vi "Data output .vi"(0 "Cluster in":refnum<vi>, 1 "Knob Refnum":refnum<vi>, 2 "Output data format":T1(ring), 5 "Pict Refnum":refnum<vi>, 7 "Clust Refnum in":refnum<vi>, 9 "Clust Refnum 3":refnum<vi>, 12 "String":string, 13 "Gyro rande \n(deg/sec)":T2(ring), 14 "Accel range \n(g)":enum16{"2", "4", "6", "8", "10", "15", "40"}(ring)) -> (3 "Gauge":i32(knob) scale=0.0..360.0, 4 "2D Picture":picture, 6 "Cluster":T5 {"Altitude" format="%#_11g"; "Longitude" format="%#_11g"; "Latitude" format="%#_11g"}, 8 "Sensors":T3 {"Altitude" format="%#_11g"; "Longitude" format="%#_11g"; "Latitude" format="%#_11g"}, 10 "QPVT":T4 {"Altitude" format="%#_11g"; "Longitude" format="%#_11g"; "Latitude" format="%#_11g"})   [LabVIEW 2017, in "IL Driver Library.lvlib"]
uses:
  IL Driver library.lvlib
panel:
  # "Orientation angles (deg)"
  # "Sensors output\n(ADC code)"
  # "Rate"
  # "Accel"
  # "Magn"
  # "X"
  # "Y"
  # "Z"
  # "Additional\n   (code)"
  # "Position abs (deg,m)"
  # "Quaternion of orientation"
  # "Sensors output"
  # "Rate(deg/s)"
  # "Accel(g)"
  # "Magn(nT)"
  # "X"
  # "Y"
  # "Z"
  # "Additional"
  # "Position abs (deg,m)"
  # "Orientation angles (deg)"
  # "Sensors output"
  # "Rate(deg/s)"
  # "Accel(g)"
  # "Magn(nT)"
  # "X"
  # "Y"
  # "Z"
  # "Additional"
  # "Position abs (deg,m)"
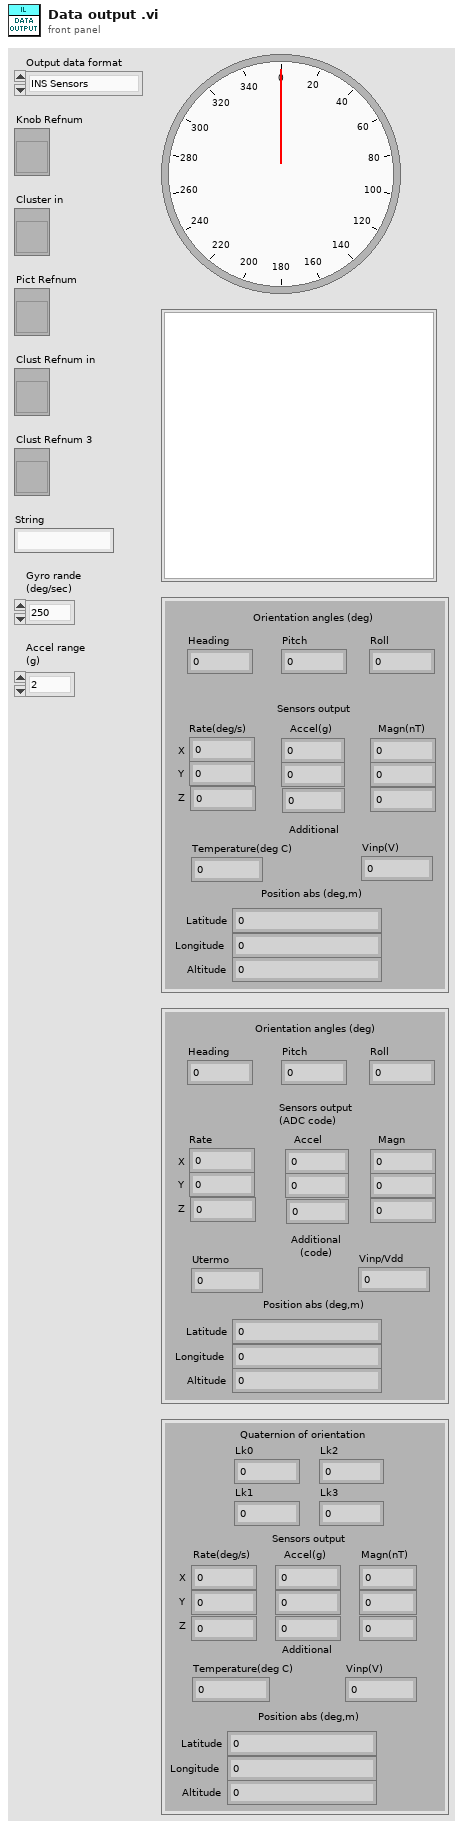
[diagram p1: front panel]
types:
  T1 = enum16{"INS Sensors", "INS OPVT", "INS QPVT", "INS OPVT2A", "INS OPVT2AW", "INS OPVT2Ahr", "INS Minimal", "INS NMEA"}
  T2 = enum16{"250", "300", "450", "500", "1000", "2000"}
  T3 = cluster{"Heading":dbl, "Pitch":dbl, "Roll":dbl, "GyroX(deg/s)":dbl, "GyroY(deg/s)":dbl, "GyroZ(deg/s)":dbl, "AxelX(g)":dbl, "AxelY(g)":dbl, "AxelZ(g)":dbl, "Dec":i32, "MagY":i32, "MagZ":i32, "Utermo":dbl, "Vinp/Vdd":dbl, "Latitude":dbl, "Longitude":dbl, "Altitude":dbl}
  T4 = cluster{"Lk0":dbl, "Lk1":dbl, "Lk2":dbl, "Lk3":dbl, "Numeric 5":dbl, "Numeric 6":dbl, "Numeric 7":dbl, "Numeric 8":dbl, "Numeric 9":dbl, "Numeric 10":dbl, i32, i32, i32, "Temperature(deg C)":dbl, "Vinp(V)":dbl, "Latitude":dbl, "Longitude":dbl, "Altitude":dbl}
  T5 = cluster{"Heading":dbl, "Pitch":dbl, "Roll":dbl, "GyroX(deg/s)":dbl, "GyroY(deg/s)":dbl, "GyroZ(deg/s)":dbl, "AxelX(g)":dbl, "AxelY(g)":dbl, "AxelZ(g)":dbl, "Dec":i32, "MagY":i32, "MagZ":i32, "Temperature(deg C)":dbl, "Vinp(V)":dbl, "Latitude":dbl, "Longitude":dbl, "Altitude":dbl}
  T6 = cluster{dbl, dbl, dbl, "Dec":i16, "Dec":i16, "Dec":i16, "Dec":i16, "Dec":i16, "Dec":i16, "Dec":i16, "Dec":i16, "Dec":i16, "Dec":i16, dbl, "Dec":u16, "Dec":u16, "Dec":i16, dbl, dbl, dbl, dbl, dbl, dbl, dbl, dbl, dbl, "Dec":i32, "Dec":u8, "Dec":u8, "Dec":u8, "Dec":u8, "Dec":u8, "Dec":u8, "Dec":u8, "Dec":u8, "Dec":u8, "Dec":u8, "Dec":u8, "Dec":u8, "Dec":u16, "Dec":u16, "Dec":u8, "Dec":u8}
  T7 = cluster{dbl, dbl, dbl, dbl, dbl, dbl, dbl, dbl, dbl, i32, i32, i32, "Dec":u16, dbl, dbl, dbl, dbl, dbl, dbl, dbl, dbl, dbl, dbl, dbl, dbl, dbl, dbl, "Dec":i32, "Dec":u8, "Dec":u8, "Dec":u8, dbl, "Dec":u16, dbl, "Dec":u8}
  T8 = cluster{dbl, dbl, dbl, dbl, dbl, dbl, dbl, dbl, dbl, dbl, i32, i32, i32, "Dec":u16, dbl, dbl, dbl, dbl, dbl, dbl, dbl, dbl, dbl, dbl, dbl, dbl, dbl, dbl, "Dec":i32, "Dec":u8, "Dec":u8, "Dec":u8, dbl, "Dec":u16, dbl, "Dec":u8}
  T9 = cluster{dbl, dbl, dbl, dbl, dbl, dbl, dbl, dbl, dbl, dbl, i32, i32, i32, dbl, dbl, dbl, dbl, dbl}
  T10 = cluster{dbl, dbl, "Roll":dbl, dbl, dbl, dbl, dbl, dbl, dbl, i16, i16, i16, "Dec":u16, dbl, dbl, dbl, dbl, dbl, dbl, dbl, dbl, dbl, dbl, dbl, dbl, dbl, dbl, "Dec":i32, "Dec":u8, "Dec":u8, "Dec":u8, dbl, "Angles position type":u8, "Heading GNSS":dbl, "Pitch GNSS":dbl, "Heading STD GNSS":dbl, "Pitch STD GNSS":dbl, "P_bar":u16, "H_bar":dbl, "New GPS":u8}
  T11 = cluster{dbl, dbl, dbl, dbl, dbl, dbl, dbl, dbl, dbl, i32, i32, i32, "Dec":u16, dbl, "Temper":dbl, dbl, dbl, dbl, dbl, dbl, dbl, dbl, dbl, dbl, dbl, dbl, dbl, "Dec":i32, "Dec":u8, "Dec":u8, "Dec":u8, dbl, "Angles position type":u8, "Heading GNSS":dbl, "Pitch GNSS":dbl, "Heading STD GNSS":dbl, "Pitch STD GNSS":dbl, "P_bar":u16, "H_bar":dbl, "New GPS":u8, "Dec":u16}
  T12 = cluster{dbl, dbl, dbl, dbl, dbl, dbl, dbl, dbl, dbl, i16, i16, i16, "Dec":u16, dbl, dbl, dbl, dbl, dbl, dbl, dbl, dbl, dbl, dbl, dbl, dbl, dbl, dbl, "Dec":i32, "Dec":u8, "Dec":u8, "Dec":u8, dbl, "Dec":u8, dbl, dbl, dbl, dbl, u16, dbl, "Dec":u8}
  T13 = cluster{"Heading":dbl, "Pitch":dbl, "Roll":dbl, "USW":u16, "Vinp":dbl, "Temper":dbl, "Latitude":dbl, "Longitude":dbl, "Altitude or Heave":dbl, "East speed":dbl, "North speed":dbl, "Vertical speed":dbl, "ms_gps":i32, "GNSS_info1":u8, "#SolnSVs":u8}
  T14 = cluster{"H":dbl, "P":dbl, "R":dbl, "Dec":dbl, "Dec":dbl, "Dec":dbl, "Dec":dbl, "Dec":dbl, "Dec":dbl, "Dec":i32, "Dec":i32, "Dec":i32, "Temperature":dbl, "Voltag":dbl, "Lat":dbl, "Long":dbl, "Alt":dbl}
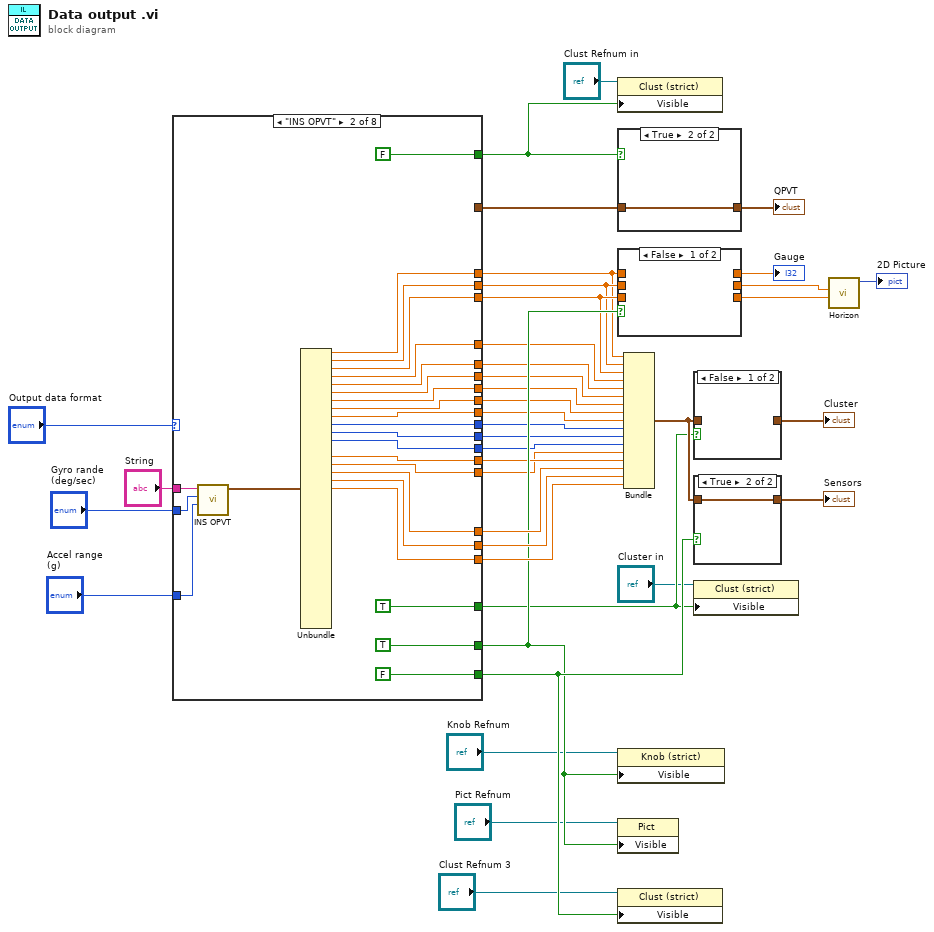
[diagram p0: block diagram]
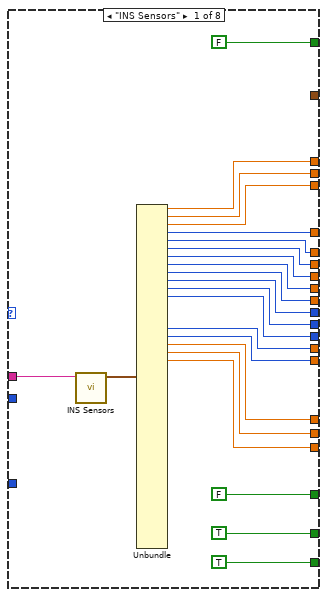
[diagram p6: hidden frame]
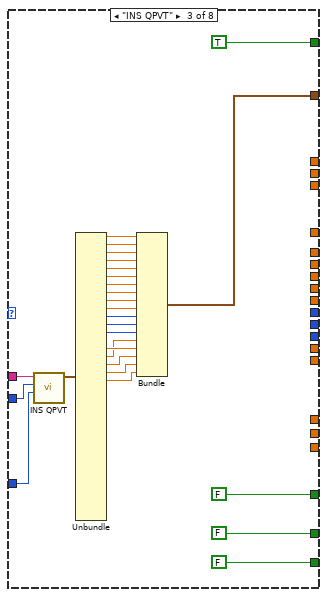
[diagram p7: hidden frame]
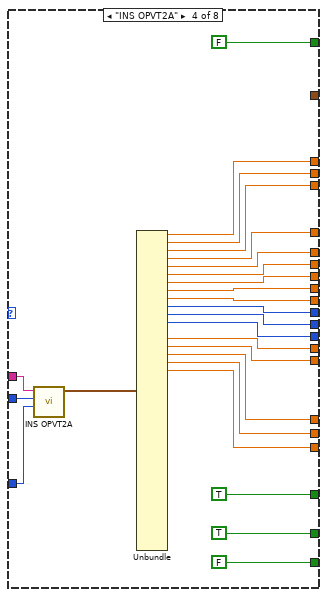
[diagram p8: hidden frame]
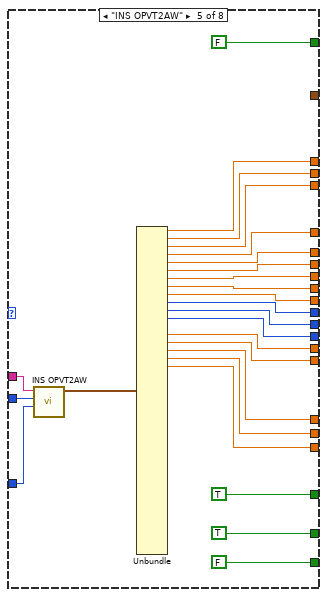
[diagram p9: hidden frame]
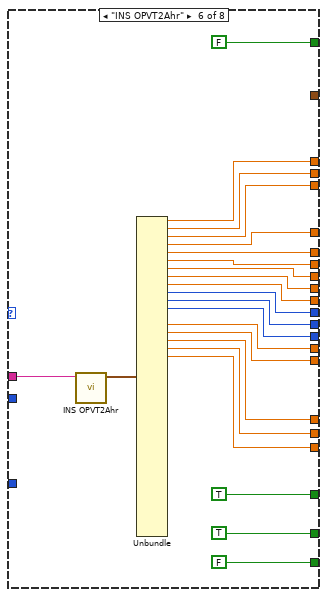
[diagram p10: hidden frame]
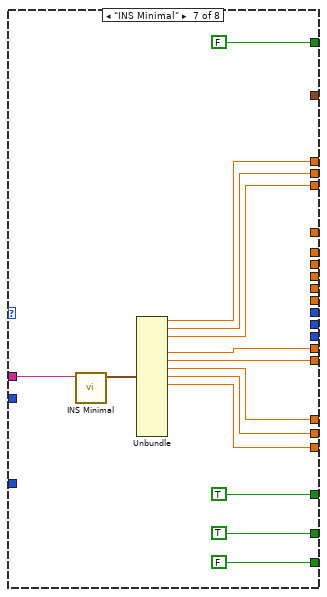
[diagram p11: hidden frame]
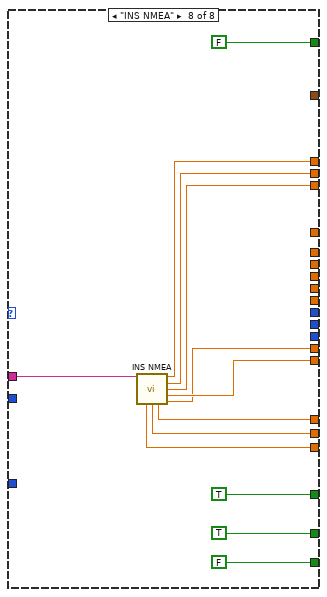
[diagram p12: hidden frame]
diagram:
  n1 = case shown="\"INS OPVT\"" "Output data format" {
    tunnel: "String" -> [w62 w73 w113 w139 w164 w173 w201 w214]
    tunnel: [w58 w87 _ w137 w162 w187 w199 w213] -> w8
    tunnel: [w60 w86 _ w136 w161 w186 w198 w212] -> w9
    tunnel: [w59 w85 _ w135 w160 w185 w197 w211] -> w10
    tunnel: [w57 w84 _ w134 w159 w184 _ _] -> w11
    tunnel: [w56 w83 _ w133 w158 w183 _ _] -> w12
    tunnel: [w55 w82 _ w132 w157 w182 _ _] -> w13
    tunnel: [w54 w81 _ w131 w156 w181 _ _] -> w14
    tunnel: [w53 w80 _ w130 w155 w180 _ _] -> w15
    tunnel: [w52 w79 _ w129 w154 w179 _ _] -> w16
    tunnel: [w51 w78 _ w128 w153 w178 _ _] -> w17
    tunnel: [w50 w77 _ w127 w152 w177 _ _] -> w18
    tunnel: [w49 w76 _ w126 w151 w176 _ _] -> w19
    tunnel: [w47 w74 _ w124 w150 w174 w195 w210] -> w20
    tunnel: [w48 w75 _ w125 w149 w175 w196 w209] -> w21
    tunnel: "Gyro rande \n(deg/sec)" -> [_ w71 w111 w123 w148 _ _ _]
    tunnel: "Accel range \n(g)" -> [_ w70 w112 w122 w147 _ _ _]
    tunnel: [FALSE TRUE FALSE TRUE TRUE TRUE TRUE TRUE] -> w26
    tunnel: [FALSE FALSE TRUE FALSE FALSE FALSE FALSE FALSE] -> w31
    tunnel: [_ _ w93 _ _ _ _ _] -> w24
    tunnel: [TRUE FALSE FALSE FALSE FALSE FALSE FALSE FALSE] -> w39
    tunnel: [TRUE TRUE FALSE TRUE TRUE TRUE TRUE TRUE] -> w34
    tunnel: [w42 w65 _ w117 w142 w168 w190 w204] -> w35
    tunnel: [w41 w64 _ w116 w141 w166 w189 w203] -> w36
    tunnel: [w40 w63 _ w115 w140 w165 w188 w202] -> w37
    frame "INS Sensors" {
      n2 = call "INS Sensors.vi"("Hex"=w62) -> ("Cluster"=w61:T6)  [unwired: 10 in]
      n3 = Unbundle(w61) -> (w58:dbl, w60:dbl, w59:dbl, "Dec"=w57:i16, "Dec"=w56:i16, "Dec"=w55:i16, "Dec"=w54:i16, "Dec"=w53:i16, "Dec"=w52:i16, "Dec"=w51:i16, "Dec"=w50:i16, "Dec"=w49:i16, "Dec"=w48:u16, "Dec"=w47:i16, w42:dbl, w41:dbl, w40:dbl)  [unwired: 26 out]
    }
    frame "INS OPVT" {
      n4 = call "INS OPVT.vi"("Accelerometer range"=w70, "Gyro rande"=w71, "Hex"=w73) -> ("Cluster"=w72:T7)  [unwired: 8 in]
      n5 = Unbundle(w72) -> (w87:dbl, w86:dbl, w85:dbl, w84:dbl, w83:dbl, w82:dbl, w81:dbl, w80:dbl, w79:dbl, w78:i32, w77:i32, w76:i32, w75:dbl, w74:dbl, w65:dbl, w64:dbl, w63:dbl)  [unwired: 18 out]
    }
    frame "INS QPVT" {
      n6 = call "INS QPVT.vi"("Accelerometer range"=w112, "Gyro rande"=w111, "Hex"=w113) -> ("Cluster"=w114:T8)  [unwired: 5 in, 3 out]
      n7 = Unbundle(w114) -> (w108:dbl, w107:dbl, w106:dbl, w105:dbl, w104:dbl, w103:dbl, w102:dbl, w101:dbl, w100:dbl, w99:dbl, w98:i32, w97:i32, w96:i32, w95:dbl, w94:dbl, w90:dbl, w89:dbl, w88:dbl)  [unwired: 18 out]
      n8 = Bundle(w108, w107, w106, w105, w104, w103, w102, w101, w100, w99, w98, w97, w96, w94, w95, w90, w89, w88) -> (w93:T9)  [unwired: 1 in]
    }
    frame "INS OPVT2A" {
      n9 = call "INS OPVT2A.vi"("Accelerometer range"=w122, "Gyro rande"=w123, "Hex"=w139) -> ("Cluster"=w138:T10)  [unwired: 8 in]
      n10 = Unbundle(w138) -> (w137:dbl, w136:dbl, "Roll"=w135:dbl, w134:dbl, w133:dbl, w132:dbl, w131:dbl, w130:dbl, w129:dbl, w128:i16, w127:i16, w126:i16, w125:dbl, w124:dbl, w117:dbl, w116:dbl, w115:dbl)  [unwired: 23 out]
    }
    frame "INS OPVT2AW" {
      n11 = call "INS OPVT2AW.vi"("Accelerometer range"=w147, "Gyro rande"=w148, "Hex"=w164) -> ("Cluster"=w163:T11)  [unwired: 8 in]
      n12 = Unbundle(w163) -> (w162:dbl, w161:dbl, w160:dbl, w159:dbl, w158:dbl, w157:dbl, w156:dbl, w155:dbl, w154:dbl, w153:i32, w152:i32, w151:i32, w149:dbl, "Temper"=w150:dbl, w142:dbl, w141:dbl, w140:dbl)  [unwired: 24 out]
    }
    frame "INS OPVT2Ahr" {
      n13 = call "INS OPVT2Ahr.vi"("Hex"=w173) -> ("Cluster"=w167:T12)  [unwired: 10 in]
      n14 = Unbundle(w167) -> (w187:dbl, w186:dbl, w185:dbl, w184:dbl, w183:dbl, w182:dbl, w181:dbl, w180:dbl, w179:dbl, w178:i16, w177:i16, w176:i16, w175:dbl, w174:dbl, w168:dbl, w166:dbl, w165:dbl)  [unwired: 23 out]
    }
    frame "INS Minimal" {
      n15 = call "INS Minimal.vi"("Hex"=w201) -> ("Cluster"=w200:T13)  [unwired: 10 in]
      n16 = Unbundle(w200) -> ("Heading"=w199:dbl, "Pitch"=w198:dbl, "Roll"=w197:dbl, "Vinp"=w196:dbl, "Temper"=w195:dbl, "Latitude"=w190:dbl, "Longitude"=w189:dbl, "Altitude or Heave"=w188:dbl)  [unwired: 7 out]
    }
    frame "INS NMEA" {
      n17 = call "INS NMEA.vi"("string"=w214) -> ("H"=w213:dbl, "P"=w212:dbl, "R"=w211:dbl, "Temperature"=w210:dbl, "Alt"=w202:dbl, "Long"=w203:dbl, "Lat"=w204:dbl, "Voltag"=w209:dbl)  [unwired: 7 in]
    }
  }
  n18 = property on="Property Node" class="Clust (strict)"(reference="Clust Refnum in", "Visible"=w31) -> ()  [unwired: 1 in, 2 out]
  n19 = case shown="True" w31 {
    tunnel: [_ w215] -> w30
    tunnel: w24 -> [_ w215]
    frame False {
    }
    frame True {
    }
  }
  "QPVT" <- w30
  n20 = case shown="False" w34 {
    tunnel: w9 -> [_ w217]
    tunnel: w10 -> [_ w216]
    tunnel: w8 -> [_ w218]
    tunnel: [_ w218] -> w27
    tunnel: [_ w217] -> w28
    tunnel: [_ w216] -> w29
    frame False {
    }
    frame True {
    }
  }
  "Gauge" <- w27
  n21 = property on="Property Node" class="Knob (strict)"(reference="Knob Refnum", "Visible"=w34) -> ()  [unwired: 1 in, 2 out]
  n22 = property on="Property Node" class="Pict"(reference="Pict Refnum", "Visible"=w34) -> ()  [unwired: 1 in, 2 out]
  n23 = property on="Property Node" class="Clust (strict)"(reference="Clust Refnum 3", "Visible"=w39) -> ()  [unwired: 1 in, 2 out]
  n24 = Bundle("H"=w8, "P"=w9, "R"=w10, "Dec"=w11, "Dec"=w12, "Dec"=w13, "Dec"=w14, "Dec"=w15, "Dec"=w16, "Dec"=w17, "Dec"=w18, "Dec"=w19, "Temperature"=w20, "Voltag"=w21, "Lat"=w35, "Long"=w36, "Alt"=w37) -> (w33:T14)  [unwired: 1 in]
  n25 = case shown="False" w26 {
    tunnel: [_ w219] -> w32
    tunnel: w33 -> [_ w219]
    frame False {
    }
    frame True {
    }
  }
  "Cluster" <- w32
  n26 = case shown="True" w39 {
    tunnel: [_ w220] -> w38
    tunnel: w33 -> [_ w220]
    frame False {
    }
    frame True {
    }
  }
  "Sensors" <- w38
  n27 = property on="Property Node" class="Clust (strict)"(reference="Cluster in", "Visible"=w26) -> ()  [unwired: 1 in, 2 out]
  n28 = call "Horizon.vi"("Roll"=w29, "Pitch"=w28) -> ("2D Picture"=→"2D Picture":picture)  [unwired: 9 in]
